vi "UHR-Fleezers Control (fpga) FB changed Ronen - 10.3.vi"() -> ()   [LabVIEW 2013]
doc: "UHR-Fleezers Instrument Control Code (fpga)"
uses:
  <vilib>/eio/EIONode/EIONode.xnode
  <vilib>/eio/EIOMethodNode/EIOMethodNode.xnode
  <vilib>/rvi/DataTransferAndStorage/Container/XNode/niFpgaContainer.xnode
  <vilib>/Platform/TimedLoop/XDataNode/XDataNode.xnode
  <vilib>/Platform/TimedLoop/XDataNode/nitl_modes.ctl
  <vilib>/Platform/TimedLoop/XDataNode/XDNodeRunTimeDep.lvlib
  <vilib>/Platform/TimedLoop/XDataNode/wakeup.ctl
  <vilib>/Platform/TimedLoop/XDataNode/timing_clust.ctl
  <vilib>/addons/control/pid/fpga.llb/XNode/niFpgaPID.xnode
  <vilib>/rvi/eio/common/nirviEmuTemplateMethod_errors.vi
  <vilib>/rvi/interface/RandomDataEmulation/nirviRandomDataFpgaReadWriteTemplate.vi
panel:
  out "Trap Pos FB Int-Norm Signal":fxp<+/-,24,9> format="%.16g"
  out "Trap Pos FB Int Signal":fxp<+/-,24,9> format="%.18g"
  in  "Tab Control":T1(tab)
  in  "AI1 X Scale":u16
  in  "Trap Pos FB Monitor T1 or T2":bool
  in  "Trap Pos FB Negate Action":bool
  in  "Trap Pos. FB SP":fxp<+/-,16,1>
  in  "Trap Pos. FB Reset":bool
  in  "Trap Pos to FIFO":bool
  in  "AI1 Sets to FIFO":T2={"Set 1"=TRUE, "Set 2"=TRUE, "Set 3"=FALSE}
  in  "N of AI1 Int Acq Sets":i16=2 min=1 max=3 step=1
  out "AI Late Counter":u16
  in  "ai count":u32=400
  out "AI late?":bool
  in  "+ phase":bool
  in  "Phase count adjustment":i16
  out "Relative phase":i16
  in  "AI to FIFO":bool
  out "BD1 Frequency Out 1":u64
  out "BD1 Frequency Out 2":u64
  in  "Force feedback":bool
  out "AI1 X Set 1":fxp<+/-,16,1>
  in  "Trap Pos. FB Gains":T3={"proportional gain (Kc)"=0.0, "integral gain (Kc*Ts/Ti)"=10.0, "derivative gain (Kc*Td/Ts)"=0.0} {"proportional gain (Kc)" format="%.11g"; "integral gain (Kc*Ts/Ti)" format="%.11g"; "derivative gain (Kc*Td/Ts)" format="%.11g"}
  in  "Trap Pos. FB Range":T4={"output high"=0.999969482421875, "output low"=-1.0}
  in  "Trap Pos. FB Mult Factor":i64=2
  in  "Trap Pos. FB Offset Factor":i64
  out "AI1 X Set 2":fxp<+/-,16,1>
  out "Trap Pos FB Action":i64
  out "Trap Pos FIFO Timeout":u16
  out "Trap AI FIFO Timeout":u16
  in  "Trap FIFO Set Timeout":i32
  in  "Trap Pos FB Int Count":u16=100
  in  "Dynamic Force FB (Ronen)":bool
  in  "Tab Control 2":T5(tab)
  in  "FB Min Frequency":u64
  in  "FB Max Frequency":u64
  in  "Negate Diff?":bool
  in  "B factor":fxp<+/-,16,16>
  in  "Diff FB Measurement?":bool
  in  "Swap F1 and F2":bool
  in  "Freq or Amp switch first":bool=TRUE
  in  "Cont. Scan":bool
  in  "Abort scan":bool
  in  "Cycles per step":u64
  in  "Scan BD":bool
  in  "Number of scans":u16
  in  "Scan steps":u64
  in  "Scan freq.  increment":i64
  out "Scanning":bool
  in  "Start scan":bool
  in  "OSK Bd 1":bool
  in  "Reset Bd 1":bool
  in  "RD":bool
  in  "PMODE":bool
  in  "OSK Bd 2":bool
  in  "Reset Bd 2":bool
  in  "Direct RF Box \nCommunication":bool
  in  "Data BD 2":u8 format="%08b"
  in  "Data BD 1":u8 format="%08b"
  in  "Address":u8 format="%02x"
  in  "Update Data":bool
  in  "FPGA Controls\n RF Box":bool
  in  "Number Interlace Cycles":u8=2 min=1 max=3
  in  "Interlace Off Parameters":u8=1 min=1 max=3
  in  "Interlace ON/OFF":bool
  out "DIO Relative phase":i16
  in  "Phase count adjustment (DIO)":i16
  in  "+ phase (DIO)":bool
  out "DIO Late Counter":u16
  out "DIO Late?":bool
  in  "DIO count 1 (ticks)":u32=400
  in  "DIO count 2 (ticks)":u32=400
  in  "DIO count 3 (ticks)":u32=400
  out "AI4 Y Sum Set 2":i16
  out "AI4 Y Sum Set 1":i16
  in  "FB Gains Set 1":T6={"proportional gain (Kc)"=10, "integral gain (Kc*Ts/Ti)"=5, "derivative gain (Kc*Td/Ts)"=0}
  in  "FB Setpoint Set 1":i16 min=0 step=1
  in  "FB Reset Set 1":bool
  in  "FB On/Off Set 1":bool
  in  "FB Reset Set 2":bool
  in  "FB On/Off Set 2":bool
  in  "FB Setpoint Set 2":i16 min=0 step=1
  in  "FB Gains Set 2":T6={"proportional gain (Kc)"=10, "integral gain (Kc*Ts/Ti)"=5, "derivative gain (Kc*Td/Ts)"=0}
  in  "FB output range 2":cluster{"output high":i16, "output low":i16}={"output high"=3000, "output low"=0}
  in  "FB output range 1":cluster{"output high":i16, "output low":i16}={"output high"=3000, "output low"=0}
  out "Scan I":u64
  in  "Amp switch delay":u16=5
  in  "Freq switch delay":u16
  in  "BD 2 Amplitude 1":u16
  in  "BD 1 Amplitude 1":u16
  in  "BD 2 Frequency 1":u64
  in  "BD 1 Frequency 1":u64
  in  "BD 2 Amplitude 2":u16
  in  "BD 1 Amplitude 2":u16
  in  "BD 2 Frequency 2":u64
  in  "BD 1 Frequency 2":u64
  in  "BD 2 Amplitude 3":u16
  in  "BD 1 Amplitude 3":u16
  in  "BD 2 Frequency 3":u64
  in  "BD 1 Frequency 3":u64
  out "Numeric":i32
  out "AO2 2":i16
  out "AO1 2":i16
  in  "1D or 2D Scan?":bool
  in  "Abort scan (MCL)":bool
  in  "MCL Scan Axis":bool
  in  "Cont. Scan (MCL)":bool
  out "Scan I (MCL)":u64
  in  "Number of scans (MCL)":u16
  out "Scanning MCL":bool
  in  "Scan steps (MCL)":u64
  in  "Cycles per step (MCL)":u64
  in  "Scan freq.  increment (MCL)":i16
  in  "Start scan (MCL)":bool
  in  "AO2":i16
  in  "AO1":i16
  out "MCL Late Counter":u16
  out "MCL Late?":bool
  in  "MCL count":u32=800
  out "MCL Relative Phase":i16
  in  "Phase count adjustment (MCL)":i16
  in  "+ phase (MCL)":bool
  in  "APD Gate Operating Mode":u8 max=2 step=1
  in  "Invert APD Gate":bool
  in  "APD Gate OFF Count":u32=100
  in  "APD Gate ON Count":u32=300
  out "APD 1 Gate Late Counter":u16
  out "APD 1 Gate Late?":bool
  out "APD 1 Gate Relative Phase":i16
  in  "Phase count adjustment (APD 1 Gate)":i16
  in  "+ phase (APD 1 Gate)":bool
  out "APD 2 Counts 0":u32
  out "APD 2 Counts 1":u32
  out "APD 1 Counts 0":u32
  out "APD 1 Counts 1":u32
  out "APD1 out state":bool
  in  "APD 2 AO scale factor":i16=1
  in  "APD 1 AO scale factor":i16=1
  in  "APD to FIFO":bool
  in  "APD Acq Rate Count":u32=20000000
  out "APD Acq Late Counter":u16
  out "APD Acq Late?":bool
  out "APD Acq Relative Phase":i16
  in  "Phase Count Adjustment (APD Acq)":i16
  in  "+ phase (APD Acq)":bool
  in  "Phase count adjustment (APD 2 Gate)":i16
  out "APD 2 Gate Late Counter":u16
  out "APD 2 Gate Late?":bool
  out "APD 2 Gate Relative Phase":i16
  in  "+ phase (APD 2 Gate)":bool
  out "APD2 out state":bool
  in  "Green Filter Flipper":bool
  out "Green FB Signals":T7
  in  "Green FB Count":u32=1200
  out "Green Late Counter":u16
  out "Green FB Late?":bool
  out "Green FB Relative Phase":i16
  in  "Phase count adjustment (Green FB)":i16=10
  in  "+ phase (Green FB)":bool
  out "Green FB Sum":i16
  in  "Green int current ON count adj":u32=150
  in  "Current Out":u16=30000
  in  "Green FB On/Off":bool
  in  "Green FB Setpoint":i16=250 min=0 step=1
  in  "Green FB Gains":T6={"proportional gain (Kc)"=10, "integral gain (Kc*Ts/Ti)"=5, "derivative gain (Kc*Td/Ts)"=0}
  in  "Green FB Reset":bool
  in  "Operating Mode 2":u8=2 max=2 step=1
  in  "Invert GI 2":bool
  in  "Green interlace OFF count 2":u32=900
  in  "Green interlace ON count 2":u32=300
  out "GI Late Counter 2":u16
  out "GI Late? 2":bool
  out "GI Relative phase 2":i16
  in  "Phase count adjustment (GI) 2":i16=20
  in  "+ phase (GI) 2":bool
  in  "Green interlace OFF count":u32=100
  out "GI Relative phase":i16
  in  "Phase count adjustment (GI)":i16
  in  "+ phase (GI)":bool
  out "GI Late?":bool
  in  "Green interlace ON count":u32=300
  out "GI Late Counter":u16
  in  "Invert GI":bool
  in  "Operating Mode":u8 max=2 step=1
  in  "Chassis2/Mod4/AO1":u16
  # "Only one of these can be on\nat a time:"
  # "Raster Scan AOD"
  # "1 (X)"
  # "2 (Y)"
  # "IR Intensity Feedback (RF BD 1)"
  # "AO1 (Y)"
  # "2D"
  # "1D"
  # "AO2 (X)"
  # "APD AO for aligning"
  # "Detection Loop"
  # "Green fluorescent laser digital gate interlacing loop"
  # "0 Forced ON\n1 Forced OFF\n2 Interlacing"
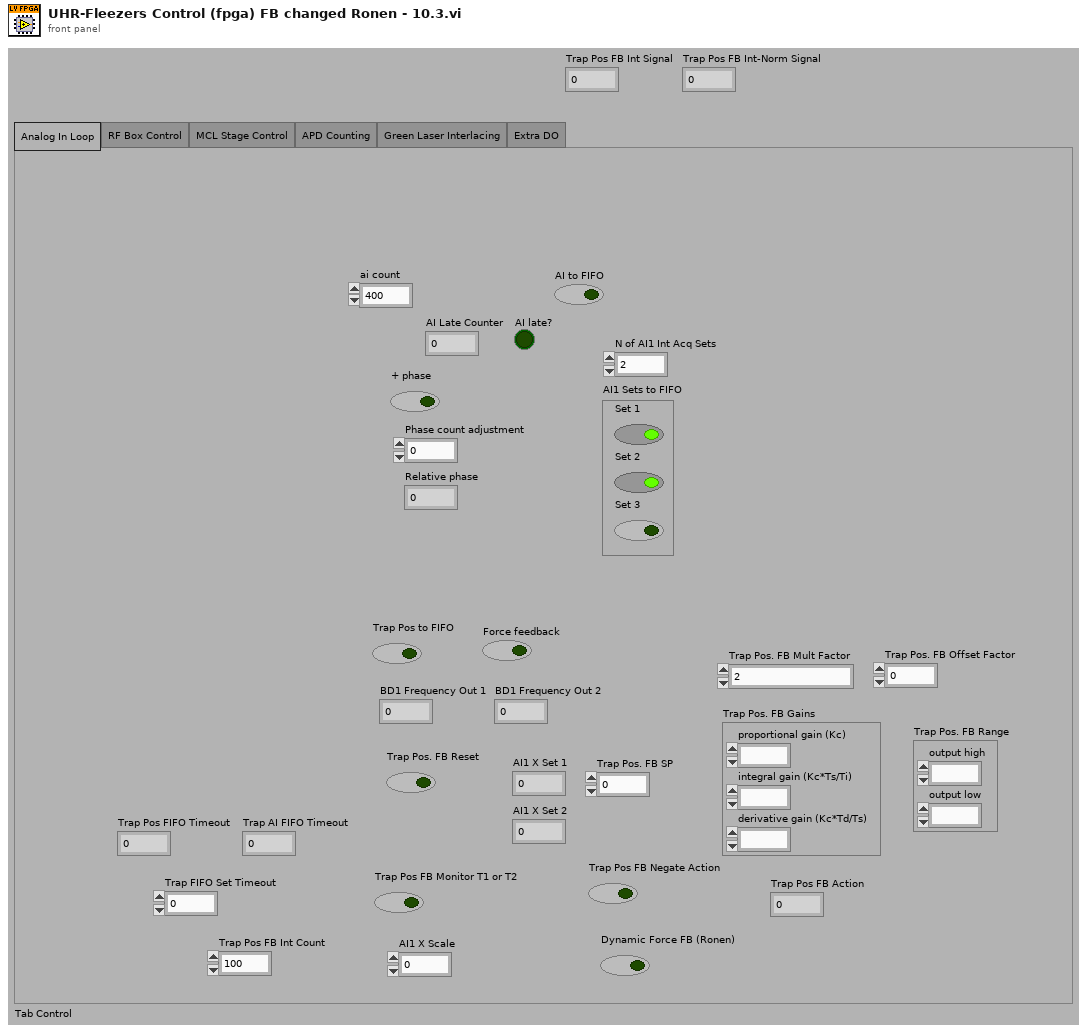
[diagram p1: front panel]
types:
  T1 = enum32{"Analog In Loop", "RF Box Control", "MCL Stage Control", "APD Counting", "Green Laser Interlacing", "Extra DO"}
  T2 = cluster{"Set 1":bool, "Set 2":bool, "Set 3":bool}
  T3 = cluster{"proportional gain (Kc)":fxp<+/-,16,8>, "integral gain (Kc*Ts/Ti)":fxp<+/-,16,8>, "derivative gain (Kc*Td/Ts)":fxp<+/-,16,8>}
  T4 = cluster{"output high":fxp<+/-,16,1>, "output low":fxp<+/-,16,1>}
  T5 = enum32{"Controls", "Interlacing Frequency and Amplitude Values"}
  T6 = cluster{"proportional gain (Kc)":i16, "integral gain (Kc*Ts/Ti)":i16, "derivative gain (Kc*Td/Ts)":i16}
  T7 = cluster{"Green FB Ch 0":i16, "Green FB Ch 1":i16, "Green FB Ch 2":i16}
  T8 = typedef "XDNodeRunTimeDep.lvlib/timing_clust.ctl" = cluster{"Expected End [f-1]":u64, "Actual End [f-1]":u64, "Finished Late? [f-1]":bool, "Expected End [i-1]":u64, "Actual End [i-1]":u64, "Finished Late? [i-1]":bool, "Expected Start [i]":u64, "Actual Start [i]":u64, "Expected Start [f]":u64, "Actual Start [f]":u64, "Source Name":string, "Structure Name":string, "Period":i64, "Deadline":i64, "Offset":i64, "Start":i64, "Priority":i32, "Timeout":i32, "Mode":T9, "Wakeup Reason":T10, "Error":errorcluster, "Source Type":string, "Secondary Source Type":string, "Global End Time":u64, "Global Start Time":u64, "Frame Duration":u64, "Iteration Duration":u64, "Assigned CPU":i32, "I/O Scan Engine Mode":u32}
  T9 = typedef "XDNodeRunTimeDep.lvlib/nitl_modes.ctl" = enum32{"No Change", "Process missed periods, maintain original phase", "Discard missed periods, maintain original phase", "Process missed periods, ignore original phase", "Discard missed periods, ignore original phase"}
  T10 = typedef "XDNodeRunTimeDep.lvlib/wakeup.ctl" = enum32{"Normal", "Aborted", "Asynchronous wakeup", "Timing source error", "Timed loop error", "Timeout"}
  T11 = cluster{"Chassis2/Mod2/AI0":i16, "Chassis2/Mod2/AI1":i16, "Chassis2/Mod2/AI2":i16}
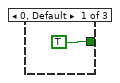
[diagram p2: hidden frame]
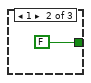
[diagram p3: hidden frame]
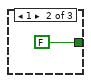
[diagram p5: hidden frame]
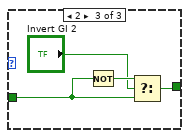
[diagram p6: hidden frame]
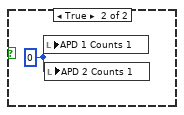
[diagram p7: hidden frame]
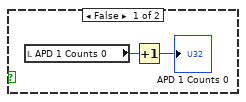
[diagram p9: hidden frame]
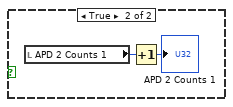
[diagram p10: hidden frame]
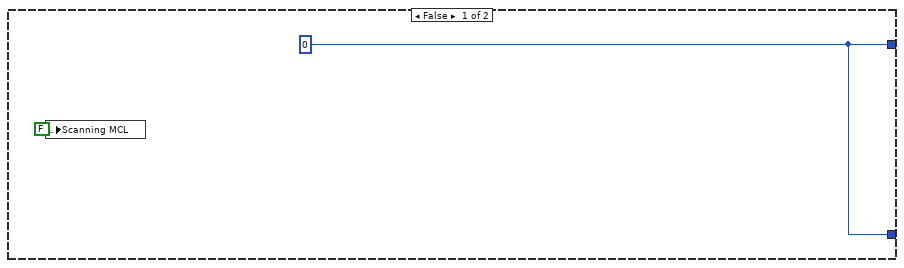
[diagram p11: hidden frame]
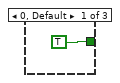
[diagram p12: hidden frame]
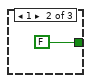
[diagram p13: hidden frame]
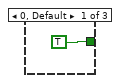
[diagram p14: hidden frame]
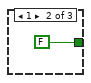
[diagram p15: hidden frame]
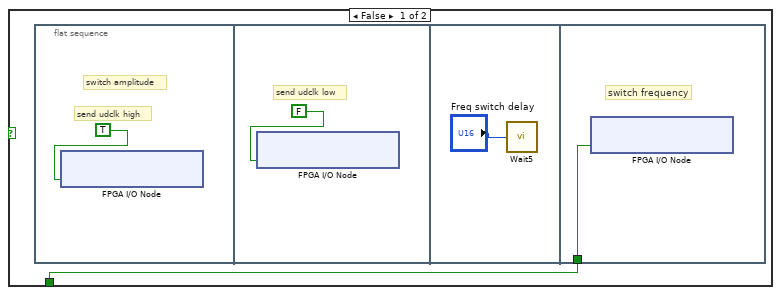
[diagram p18: hidden frame]
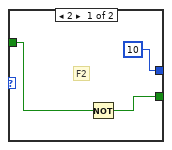
[diagram p20: hidden frame]
diagram:
  w4 = FALSE
  # "timing array current index"
  # "timing array"
  # "timing counter (phase adjusted here)"
  # "late counter"
  n1 = flat-sequence "FPGA initialization to do before running any of the loops" {
    tunnel: [u32 0 ("DIO count 3 (ticks)")] -> w3
    tunnel: [w11] -> _
    frame #0 {
      # "Start up expansion chassis early\nto avoid delays later"
      # "This pin controls udclk on the RF boards.\nWhen initially configuring the boards, this pin needs to be\nconfigured as a high impedance input.  Later it will be switched\nto an output."
      # "Initial setting of DIO data and \naddress to low (before reset).  \nThis needs to happen before the other\ncontrol method loops execute."
      n2 = xnode "FPGA I/O Node"("Connector1/DIO0"=FALSE, "Connector1/DIO1"=FALSE, "Connector1/DIO2"=FALSE, "Connector1/DIO3"=FALSE, "Connector1/DIO4"=FALSE, "Connector1/DIO5"=FALSE, "Connector1/DIO6"=FALSE, "Connector1/DIO7"=FALSE, "Connector1/DIO8"=FALSE, "Connector1/DIO9"=FALSE, "Connector1/DIO10"=FALSE, "Connector1/DIO11"=FALSE, "Connector1/DIO12"=FALSE, "Connector1/DIO13"=FALSE, "Connector1/DIO15"=FALSE, "Connector1/DIO20"=FALSE, "Connector1/DIO21"=FALSE, "Connector1/DIO22"=FALSE, "Connector1/DIO23"=FALSE, "Connector1/DIO24"=FALSE, "Connector1/DIO25"=FALSE, "Connector1/DIO26"=FALSE, "Connector1/DIO27"=FALSE, "Connector1/DIO14"=FALSE) -> ()  [unwired: 24 in, 24 out]
      n3 = xnode "FPGA I/O Method Node"("Enable"=FALSE) -> ()  [unwired: 1 in, 1 out]
      n4 = xnode "FPGA I/O Node"("Chassis2/Mod1/AO0"=u16 0 ("Chassis2/Mod4/AO0")) -> ("Chassis2/Mod2/AI0"=w11:i16)  [unwired: 2 in, 2 out]
    }
  }
  n5 = local read "AO1"() -> (w8:i16)
  n6 = local read "AO2"() -> (w7:i16)
  n7 = node-c288() -> (w6:T8)  [unwired: 1 in]
  n8 = while "APD 1 Counter" {
    tunnel: w3 -> [_]
    stop <- FALSE stop-if-true
    n9 = flat-sequence {
      frame #0 {
        n10 = xnode "FPGA I/O Method Node"("FPGA I/O In"=refnum<k21> "Connector0/DIO0" ("APD 1 DO"), "Timeout"=-1) -> ()  [unwired: 2 out]
      }
      frame #1 {
        n11 = local read "APD1 out state"() -> (w42:bool)
        n12 = case shown="True" w42 {
          frame False {
            n13 = local read "APD 1 Counts 0"() -> (w44:u32)
            n14 = Increment(x=w44) -> (x+1=→"APD 1 Counts 0":u32)
          }
          frame True {
            n15 = local read "APD 1 Counts 1"() -> (w46:u32)
            n16 = Increment(x=w46) -> (x+1=→"APD 1 Counts 1":u32)
          }
        }
      }
    }
  }
  n17 = while "APD 2 Counter" {
    tunnel: w3 -> [_]
    stop <- FALSE stop-if-true
    n18 = flat-sequence {
      frame #0 {
        n19 = xnode "FPGA I/O Method Node"("FPGA I/O In"=refnum<k21> "Connector0/DIO1" ("APD 2 DO"), "Timeout"=-1) -> ()  [unwired: 2 out]
      }
      frame #1 {
        n20 = local read "APD2 out state"() -> (w50:bool)
        n21 = case shown="False" w50 {
          frame False {
            n22 = local read "APD 2 Counts 0"() -> (w52:u32)
            n23 = Increment(x=w52) -> (x+1=→"APD 2 Counts 0":u32)
          }
          frame True {
            n24 = local read "APD 2 Counts 1"() -> (w54:u32)
            n25 = Increment(x=w54) -> (x+1=→"APD 2 Counts 1":u32)
          }
        }
      }
    }
  }
  n26 = timed-loop "RF box board DIO control: control bits" {
    timing: w6 -> [_]
    timing-out: [_] -> w5
    tunnel: [w55] -> _
    tunnel: w3 -> [w55]
    stop <- FALSE stop-if-true
    n27 = xnode "FPGA I/O Node"("Connector1/DIO16"="RD", "Connector1/DIO17"="PMODE", "Connector1/DIO18"="OSK Bd 1", "Connector1/DIO19"="Reset Bd 1", "Connector1/DIO28"="OSK Bd 2", "Connector1/DIO29"="Reset Bd 2") -> ()  [unwired: 6 in, 6 out]
  }
  n28 = while "Control Additional IO (Green laser flip mount)" {
    stop <- FALSE stop-if-true
    n29 = xnode "FPGA I/O Node"("Connector0/DIO3"="Green Filter Flipper", "Chassis2/Mod1/AO1"="Chassis2/Mod4/AO1") -> ()  [unwired: 2 in, 2 out]
    n30 = call "Loop Timer2"("Count(Ticks)"=u32 40000 ("Extra DO Counts")) -> ()  [unwired: 1 out]
  }
  n31 = while "RF box board direct communication loop" {
    tunnel: w3 -> [_]
    stop <- FALSE stop-if-true
    n32 = case "Whether to use direct communication method (only use one method at a time)" shown="True" "Direct RF Box \nCommunication" {
      frame False {
      }
      frame True {
        n33 = case shown="True" "Update Data" {
          frame False {
          }
          frame True {
            n34 = flat-sequence {
              frame #0 {
                n35 = First Call?() -> (First Call?: T/F=w72:bool)
                n36 = case shown="True" w72 {
                  frame False {
                  }
                  frame True {
                    # "If first time data updated, be sure to set WR high\nbefore setting data and address bits."
                    n37 = flat-sequence {
                      frame #0 {
                        n38 = xnode "FPGA I/O Node"("Connector1/DIO15"=TRUE) -> ()  [unwired: 1 in, 1 out]
                      }
                      frame #1 {
                        n39 = call "Wait"("Count(Ticks)"=u8 40 ("DO Delay 3 (Ticks)")) -> ()  [unwired: 1 out]
                      }
                    }
                  }
                }
              }
              frame #1 {
                n40 = Number To Boolean Array(number="Address") -> (Boolean array=w121:bool[])
                n41 = Number To Boolean Array(number="Data BD 1") -> (Boolean array=w122:bool[])
                n42 = Number To Boolean Array(number="Data BD 2") -> (Boolean array=w91:bool[])
                n43 = Index Array(array=w122, index=7) -> (element=w106:bool)
                n44 = Index Array(array=w122, index=6) -> (element=w105:bool)
                n45 = Index Array(array=w122, index=5) -> (element=w104:bool)
                n46 = Index Array(array=w122, index=4) -> (element=w103:bool)
                n47 = Index Array(array=w122, index=3) -> (element=w102:bool)
                n48 = Index Array(array=w122, index=2) -> (element=w101:bool)
                n49 = Index Array(array=w122, index=1) -> (element=w100:bool)
                n50 = Index Array(array=w122, index=0) -> (element=w99:bool)
                n51 = Index Array(array=w121, index=5) -> (element=w98:bool)
                n52 = Index Array(array=w121, index=4) -> (element=w97:bool)
                n53 = Index Array(array=w121, index=3) -> (element=w96:bool)
                n54 = Index Array(array=w121, index=2) -> (element=w95:bool)
                n55 = Index Array(array=w121, index=1) -> (element=w94:bool)
                n56 = Index Array(array=w121, index=0) -> (element=w93:bool)
                n57 = Index Array(array=w91, index=7) -> (element=w82:bool)
                n58 = Index Array(array=w91, index=6) -> (element=w81:bool)
                n59 = Index Array(array=w91, index=5) -> (element=w80:bool)
                n60 = Index Array(array=w91, index=4) -> (element=w79:bool)
                n61 = Index Array(array=w91, index=3) -> (element=w78:bool)
                n62 = Index Array(array=w91, index=2) -> (element=w77:bool)
                n63 = Index Array(array=w91, index=1) -> (element=w76:bool)
                n64 = Index Array(array=w91, index=0) -> (element=w75:bool)
                n65 = xnode "FPGA I/O Node"("Connector1/DIO0"=w106, "Connector1/DIO1"=w105, "Connector1/DIO2"=w104, "Connector1/DIO3"=w103, "Connector1/DIO4"=w102, "Connector1/DIO5"=w101, "Connector1/DIO6"=w100, "Connector1/DIO7"=w99, "Connector1/DIO8"=w98, "Connector1/DIO9"=w97, "Connector1/DIO10"=w96, "Connector1/DIO11"=w95, "Connector1/DIO12"=w94, "Connector1/DIO13"=w93, "Connector1/DIO20"=w82, "Connector1/DIO21"=w81, "Connector1/DIO22"=w80, "Connector1/DIO23"=w79, "Connector1/DIO24"=w78, "Connector1/DIO25"=w77, "Connector1/DIO26"=w76, "Connector1/DIO27"=w75) -> ()  [unwired: 22 in, 22 out]
              }
              frame #2 {
                # "wait and then apply write signal"
                n66 = call "Wait2"("Count(Ticks)"=u8 40 ("DO Delay 1 (Ticks)")) -> ()  [unwired: 1 out]
              }
              frame #3 {
                # "sending bit low writes data to board buffer"
                n67 = xnode "FPGA I/O Node"("Connector1/DIO15"=FALSE) -> ()  [unwired: 1 in, 1 out]
              }
              frame #4 {
                # "wait then return write signal"
                n68 = call "Wait3"("Count(Ticks)"=u8 40 ("DO Delay 2 (Ticks)")) -> ()  [unwired: 1 out]
              }
              frame #5 {
                # "sending bit high makes ready to\nwrite more data"
                n69 = xnode "FPGA I/O Node"("Connector1/DIO15"=TRUE) -> ()  [unwired: 1 in, 1 out]
              }
            }
          }
        }
      }
    }
  }
  n70 = while "APD 2 Gating" {
    shift-right: [w132] -> _
    shift-left: w3 -> [w137]
    shift-right: [w131] -> _
    shift-left: w4 -> [w129]
    stop <- FALSE stop-if-true
    n71 = flat-sequence {
      tunnel: w137 -> [w140]
      tunnel: [w141] -> w135
      tunnel: [w140] -> w133
      tunnel: [w139] -> w130
      tunnel: w129 -> [w139]
      tunnel: [w144] -> w136
      tunnel: w135 -> [w144]
      tunnel: [w143] -> w134
      tunnel: w133 -> [w143]
      tunnel: w130 -> [w142]
      tunnel: [w162] -> w132
      tunnel: w136 -> [w173]
      tunnel: w134 -> [w171]
      tunnel: [w166] -> w131
      frame #0 {
        n72 = call "Loop Timer8"("Count(Ticks)"=w140) -> ("Tick Count(Ticks)"=w141:u32)
      }
      frame #1 {
        # "(need 4 channels/APD)"
        n73 = xnode "FPGA I/O Node"("Connector1/DIO26"=w142, "Connector1/DIO27"=w142, "Connector1/DIO22"=w142, "Connector1/DIO32"=w142, "Connector1/DIO34"=w142, "Connector1/DIO33"=w142, "Connector1/DIO35"=w142) -> ()  [unwired: 7 in, 7 out]
      }
      frame #2 {
        n74 = local read "APD Gate ON Count"() -> (w155:u32)
        n75 = local read "APD Gate OFF Count"() -> (w154:u32)
        n76 = feedback #1(TRUE) -> (w168:bool)
        n77 = feedback-in #2(w173) -> ()
        n78 = feedback #2(w173) -> (w156:u32)
        n79 = Not(x=w168) -> (.not. x?=w165:bool)
        n80 = feedback-in #1(w165) -> ()
        n81 = Subtract(x=w173, y=w156) -> (x-y=w172:u32)
        n82 = Select(t=w155, s=w165, f=w154) -> (s? t:f=w170:u32)
        n83 = Subtract(x=w172, y=w171) -> (x-y=w147:u32)
        n84 = Subtract(x=w170, y=w147) -> (x-y=w161:u32)
        n85 = Number To Boolean Array(number=w147) -> (Boolean array=w146:bool[])
        n86 = Or Array Elements(Boolean array=w146) -> (logical OR=w145:bool)
        "APD 2 Gate Late?" <- w145
        n87 = Boolean To (0,1)(Boolean="+ phase (APD 2 Gate)") -> (0, 1=w159:i16)
        n88 = Multiply(x=w159, y="Phase count adjustment (APD 2 Gate)") -> (x*y=w157:i16)
        n89 = Boolean To (0,1)(Boolean=w145) -> (0, 1=w152:i16)
        n90 = Add(x=w161, y=w157) -> (x+y=w162:u32)
        n91 = To Unsigned Word Integer(number=w152) -> (unsigned 16bit integer=w149:u16)
        n92 = feedback #3(i16 0) -> (w164:i16)
        n93 = Subtract(x=w164, y=w157) -> (x-y=w163:i16)
        "APD 2 Gate Relative Phase" <- w163
        n94 = feedback-in #3(w163) -> ()
        n95 = feedback #4(u16 0) -> (w150:u16)
        n96 = Add(x=w149, y=w150) -> (x+y=w148:u16)
        "APD 2 Gate Late Counter" <- w148
        n97 = feedback-in #4(w148) -> ()
        n98 = local read "APD Gate Operating Mode"() -> (w153:u8)
        n99 = case shown="2" w153 {
          tunnel: [TRUE FALSE w179] -> w166
          tunnel: w168 -> [_ _ w177]
          frame 0, Default {
          }
          frame 1 {
          }
          frame 2 {
            n100 = local read "Invert APD Gate"() -> (w176:bool)
            n101 = Not(x=w177) -> (.not. x?=w178:bool)
            n102 = Select(t=w178, s=w176, f=w177) -> (s? t:f=w179:bool)
          }
        }
      }
    }
  }
  n103 = while "APD 1 Gating" {
    shift-right: [w183] -> _
    shift-left: w3 -> [w188]
    shift-right: [w182] -> _
    shift-left: w4 -> [w180]
    stop <- FALSE stop-if-true
    n104 = flat-sequence {
      tunnel: w188 -> [w191]
      tunnel: [w192] -> w186
      tunnel: [w191] -> w184
      tunnel: [w190] -> w181
      tunnel: w180 -> [w190]
      tunnel: [w195] -> w187
      tunnel: w186 -> [w195]
      tunnel: [w194] -> w185
      tunnel: w184 -> [w194]
      tunnel: w181 -> [w193]
      tunnel: [w209] -> w183
      tunnel: w187 -> [w224]
      tunnel: w185 -> [w221]
      tunnel: [w213] -> w182
      frame #0 {
        n105 = call "Loop Timer7"("Count(Ticks)"=w191) -> ("Tick Count(Ticks)"=w192:u32)
      }
      frame #1 {
        # "(need 4 channels/APD)"
        n106 = xnode "FPGA I/O Node"("Connector0/DIO8"=w193, "Connector0/DIO9"=w193, "Connector0/DIO10"=w193, "Connector0/DIO11"=w193, "Connector0/DIO4"=w193, "Connector0/DIO5"=w193, "Connector0/DIO6"=w193, "Connector0/DIO7"=w193) -> ()  [unwired: 8 in, 8 out]
      }
      frame #2 {
        n107 = feedback #5(TRUE) -> (w216:bool)
        n108 = feedback-in #6(w224) -> ()
        n109 = feedback #6(w224) -> (w223:u32)
        n110 = Not(x=w216) -> (.not. x?=w212:bool)
        n111 = feedback-in #5(w212) -> ()
        n112 = Subtract(x=w224, y=w223) -> (x-y=w222:u32)
        n113 = Select(t="APD Gate ON Count", s=w212, f="APD Gate OFF Count") -> (s? t:f=w218:u32)
        n114 = Subtract(x=w222, y=w221) -> (x-y=w197:u32)
        n115 = Subtract(x=w218, y=w197) -> (x-y=w208:u32)
        n116 = Number To Boolean Array(number=w197) -> (Boolean array=w198:bool[])
        n117 = Or Array Elements(Boolean array=w198) -> (logical OR=w196:bool)
        "APD 1 Gate Late?" <- w196
        n118 = Boolean To (0,1)(Boolean="+ phase (APD 1 Gate)") -> (0, 1=w206:i16)
        n119 = Boolean To (0,1)(Boolean=w196) -> (0, 1=w203:i16)
        n120 = Multiply(x=w206, y="Phase count adjustment (APD 1 Gate)") -> (x*y=w204:i16)
        n121 = To Unsigned Word Integer(number=w203) -> (unsigned 16bit integer=w200:u16)
        n122 = Add(x=w208, y=w204) -> (x+y=w209:u32)
        n123 = feedback #7(i16 0) -> (w211:i16)
        n124 = Subtract(x=w211, y=w204) -> (x-y=w210:i16)
        "APD 1 Gate Relative Phase" <- w210
        n125 = feedback-in #7(w210) -> ()
        n126 = feedback #8(u16 0) -> (w201:u16)
        n127 = Add(x=w200, y=w201) -> (x+y=w199:u16)
        "APD 1 Gate Late Counter" <- w199
        n128 = feedback-in #8(w199) -> ()
        n129 = case shown="2" "APD Gate Operating Mode" {
          tunnel: [TRUE FALSE w230] -> w213
          tunnel: w216 -> [_ _ w227]
          frame 0, Default {
          }
          frame 1 {
          }
          frame 2 {
            n130 = Not(x=w227) -> (.not. x?=w229:bool)
            n131 = Select(t=w229, s="Invert APD Gate", f=w227) -> (s? t:f=w230:bool)
          }
        }
      }
    }
  }
  n132 = while "DAQ AI set 1" {
    shift-right: [w231] -> _
    shift-left: w3 -> [w236]
    stop <- FALSE stop-if-true
    n133 = flat-sequence {
      tunnel: w236 -> [w246]
      tunnel: [w247] -> w234
      tunnel: [w246] -> w233
      tunnel: [w257] -> w244
      tunnel: [w256] -> w243
      tunnel: [w255] -> w242
      tunnel: [w254] -> w241
      tunnel: [w253] -> w240
      tunnel: [w252] -> w239
      tunnel: [w251] -> w238
      tunnel: [w250] -> w237
      tunnel: [w249] -> w235
      tunnel: w234 -> [w249]
      tunnel: w233 -> [w248]
      tunnel: [w248] -> w232
      tunnel: [w287] -> w231
      tunnel: w244 -> [w314]
      tunnel: w243 -> [w279]
      tunnel: w242 -> [w280]
      tunnel: w241 -> [w313]
      tunnel: w240 -> [w259]
      tunnel: w239 -> [w302]
      tunnel: w238 -> [w301]
      tunnel: w237 -> [w300]
      tunnel: w235 -> [w297]
      tunnel: w232 -> [w294]
      frame #0 {
        n134 = call "Loop Timer3"("Count(Ticks)"=w246) -> ("Tick Count(Ticks)"=w247:u32)
      }
      frame #1 {
        # "detection \nlaser qpd"
        # "sum"
        # "x"
        # "y"
        # "1064 int\nfeedback qpd"
        # "sum"
        # "x"
        # "traps\nqpd"
        # "sum"
        # "y"
        # "x"
        n135 = xnode "FPGA I/O Node"("Connector1/DIO31"=TRUE ("Connector1/DIO33")) -> ("Connector0/AI0"=w257:i16, "Connector0/AI1"=w256:i16, "Connector0/AI2"=w255:i16, "Connector0/AI3"=w254:i16, "Connector0/AI4"=w253:i16, "Connector0/AI5"=w252:i16, "Connector0/AI6"=w251:i16, "Connector0/AI7"=w250:i16)  [unwired: 9 in, 9 out]
      }
      frame #2 {
        w283 = FALSE ("AI to FIFO")
        # "only write specified sets (1 and 2 usually) to FIFO \nif AI to FIFO is true"
        # "Adjust phase after data acquired if button pressed"
        n136 = feedback #9(i16 1) -> (w306:i16)
        n137 = Increment(x=w306) -> (x+1=w312:i16)
        n138 = Scale By Power Of 2(n="AI1 X Scale", x=w279) -> (x*2^n=w277:i16)
        n139 = Greater?(x=w312, y="N of AI1 Int Acq Sets") -> (0:w309:bool)
        n140 = Divide(x=w277, y=w280) -> (x/y=w276:fxp<+/-,16,1>)
        n141 = Select(t=i16 1, s=w309, f=w312) -> (s? t:f=w311:i16)
        n142 = feedback-in #9(w311) -> ()
        n143 = feedback #10(w283) -> (w281:bool)
        n144 = feedback #11(w283) -> (w299:bool)
        n145 = case shown="3" w306 {
          tunnel: w259 -> [w336 w344 _]
          tunnel: "AI1 Sets to FIFO" -> [w340 w348 w354]
          tunnel: [w339 w347 w353] -> w303
          tunnel: ["AI to FIFO" w346 w352] -> w298
          tunnel: w299 -> [_ w346 w352]
          tunnel: ["Trap Pos to FIFO" w345 w351] -> w282
          tunnel: w281 -> [_ w345 w351]
          tunnel: w276 -> [w335 w343 _]
          tunnel: [w334 w341 FALSE] -> w263
          tunnel: [w333 w342 u64 0 ("BD1 Frequency Out 2")] -> w262
          frame 1, Default {
            n146 = Unbundle By Name(w340) -> ("Set 1"=w339:bool)
            n147 = local read "BD1 Frequency Out 1"() -> (w333:u64)
            n148 = Compound Arithmetic op=AND("Trap Pos to FIFO", w339, "AI to FIFO") -> (w334:bool)
            "AI4 Y Sum Set 1" <- w336
            "AI1 X Set 1" <- w335
          }
          frame 2 {
            n149 = Unbundle By Name(w348) -> ("Set 2"=w347:bool)
            n150 = local read "BD1 Frequency Out 2"() -> (w342:u64)
            n151 = Compound Arithmetic op=AND(w345, w347, w346) -> (w341:bool)
            "AI4 Y Sum Set 2" <- w344
            "AI1 X Set 2" <- w343
          }
          frame 3 {
            n152 = Unbundle By Name(w354) -> ("Set 3"=w353:bool)
          }
        }
        n153 = And(x=w303, y=w298) -> (x .and. y?=w305:bool)
        n154 = feedback-in #10(w282) -> ()
        n155 = case shown="True" w305 {
          tunnel: w314 -> [_ w368]
          tunnel: w279 -> [_ w367]
          tunnel: w280 -> [_ w366]
          tunnel: w313 -> [_ w365]
          tunnel: w259 -> [_ w364]
          tunnel: w302 -> [_ w363]
          tunnel: w301 -> [_ w362]
          tunnel: w300 -> [_ w361]
          tunnel: 0 ("DMA buffer timeout") -> [_ w370]
          frame False {
          }
          frame True {
            n156 = Build Array(w368, w367, w366, w365, w364, w363, w362, w361) -> (w369:i16[])
            n157 = for {
              tunnel: w369 -> [w372] mode=indexing
              tunnel: w370 -> [w373]
              tunnel: [w371] -> w359 mode=indexing
              n158 = xnode ("FIFO Write")("Element"=w372, "Timeout"=w373) -> ("Timed Out?"=w371:bool)  [unwired: 1 in, 1 out]
            }
            n159 = Or Array Elements(Boolean array=w359) -> (logical OR=w356:bool)
            n160 = Boolean To (0,1)(Boolean=w356) -> (0, 1=w358:i16)
            n161 = feedback #12(u16 0) -> (w357:u16)
            n162 = Add(x=w358, y=w357) -> (x+y=w355:u16)
            "Trap AI FIFO Timeout" <- w355
            n163 = feedback-in #12(w355) -> ()
          }
        }
        n164 = feedback-in #11(w298) -> ()
        n165 = case shown="True" w263 {
          tunnel: w262 -> [_ w320]
          tunnel: [u8 0 w317] -> w261
          frame False {
          }
          frame True {
            n166 = Split Number(x=w320) -> (hi(x)=w321:u32, lo(x)=w322:u32)
            n167 = Split Number(x=w321) -> (lo(x)=w323:u16)  [unwired: 1 out]
            n168 = Split Number(x=w322) -> (hi(x)=w324:u16, lo(x)=w325:u16)
            n169 = Build Array "BD 1 nu Stack"(w323, w324, w325) -> (w319:u16[])
            n170 = for {
              tunnel: w319 -> [w332] mode=indexing
              shift-right: [w328] -> w317
              shift-left: u8 0 -> [w329]
              n171 = xnode ("FIFO Method Node")("Element"=w332, "Timeout"="Trap FIFO Set Timeout") -> ("Timed Out?"=w331:bool)  [unwired: 1 in, 1 out]
              n172 = Boolean To (0,1)(Boolean=w331) -> (0, 1=w330:i16)
              n173 = To Unsigned Byte Integer(number=w330) -> (unsigned 8bit integer=w327:u8)
              n174 = Add(x=w327, y=w329) -> (x+y=w328:u8)
            }
          }
        }
        n175 = To Unsigned Word Integer(number=w261) -> (unsigned 16bit integer=w260:u16)
        n176 = feedback #13(u16 0) -> (w274:u16)
        n177 = Add(x=w260, y=w274) -> (x+y=w273:u16)
        "Trap Pos FIFO Timeout" <- w273
        n178 = feedback-in #13(w273) -> ()
        n179 = feedback-in #14(w297) -> ()
        n180 = feedback #14(w297) -> (w296:u32)
        n181 = Subtract(x=w297, y=w296) -> (x-y=w295:u32)
        n182 = xnode "I/O Node"("Connector1/DIO31"=FALSE ("Connector1/DIO34")) -> ()  [unwired: 1 in, 1 out]
        n183 = Subtract(x=w295, y=w294) -> (x-y=w265:u32)
        n184 = Boolean To (0,1)(Boolean="+ phase") -> (0, 1=w290:i16)
        n185 = Multiply(x=w290, y="Phase count adjustment") -> (x*y=w284:i16)
        n186 = Subtract(x="ai count", y=w265) -> (x-y=w288:u32)
        n187 = Number To Boolean Array(number=w265) -> (Boolean array=w266:bool[])
        n188 = feedback #15(i16 0) -> (w286:i16)
        n189 = Add(x=w288, y=w284) -> (x+y=w287:u32)
        n190 = Subtract(x=w286, y=w284) -> (x-y=w285:i16)
        "Relative phase" <- w285
        n191 = feedback-in #15(w285) -> ()
        n192 = Or Array Elements(Boolean array=w266) -> (logical OR=w264:bool)
        "AI late?" <- w264
        n193 = Boolean To (0,1)(Boolean=w264) -> (0, 1=w271:i16)
        n194 = To Unsigned Word Integer(number=w271) -> (unsigned 16bit integer=w268:u16)
        n195 = feedback #16(u16 0) -> (w269:u16)
        n196 = Add(x=w268, y=w269) -> (x+y=w267:u16)
        "AI Late Counter" <- w267
        n197 = feedback-in #16(w267) -> ()
      }
    }
  }
  n198 = while "MCL stage control" {
    shift-right: [w389] -> _
    shift-left: w3 -> [w392]
    shift-right: [w382] -> _
    shift-left: w8 -> [w379]
    shift-right: [w381] -> _
    shift-left: w7 -> [w377]
    i -> [w376]
    stop <- FALSE stop-if-true
    n199 = flat-sequence {
      tunnel: w392 -> [w396]
      tunnel: [w397] -> w388
      tunnel: [w396] -> w386
      tunnel: [w395] -> w380
      tunnel: w379 -> [w395]
      tunnel: [w394] -> w378
      tunnel: w377 -> [w394]
      tunnel: w388 -> [w401]
      tunnel: [w401] -> w387
      tunnel: w386 -> [w400]
      tunnel: [w400] -> w385
      tunnel: w380 -> [w399]
      tunnel: w378 -> [w398]
      tunnel: [w399] -> w375
      tunnel: [w398] -> w374
      tunnel: w387 -> [w411]
      tunnel: w385 -> [w410]
      tunnel: [w411] -> w391
      tunnel: [w410] -> w390
      tunnel: [w409] -> w384
      tunnel: [w408] -> w383
      tunnel: w375 -> [w403]
      tunnel: w374 -> [w402]
      tunnel: [w483] -> w389
      tunnel: w391 -> [w490]
      tunnel: w390 -> [w487]
      tunnel: w384 -> [w485]
      tunnel: w383 -> [w484]
      tunnel: [w485] -> w382
      tunnel: [w484] -> w381
      frame #0 {
        n200 = call "Loop Timer5"("Count(Ticks)"=w396) -> ("Tick Count(Ticks)"=w397:u32)
      }
      frame #1 {
        n201 = xnode "FPGA I/O Node"("Connector0/AO1"=w399, "Connector0/AO2"=w398) -> ()  [unwired: 2 in, 2 out]
      }
      frame #2 {
        n202 = local read "Scanning MCL"() -> (w423:bool)
        n203 = Or(x=w423, y="Start scan (MCL)") -> (x .or. y?=w418:bool)
        n204 = Not(x="Abort scan (MCL)") -> (.not. x?=w416:bool)
        n205 = And(x=w416, y=w418) -> (x .and. y?=w415:bool)
        n206 = case "Raster scan" shown="True" w415 {
          tunnel: [w424 w467] -> w420
          tunnel: "Start scan (MCL)" -> [_ w452]
          tunnel: [w424 w428] -> w404
          frame False {
            w424 = i16 0
            n207 = local write "Scanning MCL"(FALSE ("scanning")) -> ()
          }
          frame True {
            w438 = i16 0
            w437 = u64 0
            # "scan incr."
            # "freq. incr. mult."
            # "count steps"
            # "count number of cycles"
            n208 = feedback #17(w437) -> (w464:u64)
            n209 = Select(t=w437, s=w452, f=w464) -> (s? t:f=w466:u64)
            n210 = Increment(x=w466) -> (x+1=w463:u64)
            n211 = Greater?(x="Cycles per step (MCL)", y=w463) -> (0:w447:bool)
            n212 = Select(t=w463, s=w447, f=w437) -> (s? t:f=w462:u64)
            n213 = feedback-in #17(w462) -> ()
            n214 = feedback #18(w437) -> (w461:u64)
            n215 = Select(t=w437, s=w452, f=w461) -> (s? t:f=w456:u64)
            n216 = Increment(x=w456) -> (x+1=w460:u64)
            n217 = Add(x="Scan steps (MCL)", y="Scan steps (MCL)") -> (x+y=w459:u64)
            n218 = Select(t=w456, s=w447, f=w460) -> (s? t:f=w442:u64)
            n219 = Greater?(x=w459, y=w442) -> (0:w441:bool)
            n220 = Select(t=w442, s=w441, f=w437) -> (s? t:f=w457:u64)
            n221 = feedback-in #18(w457) -> ()
            n222 = Equal?(x="Scan steps (MCL)", y=w442) -> (x = y?=w446:bool)
            n223 = Greater?(x="Scan steps (MCL)", y=w456) -> (0:w455:bool)
            n224 = feedback #19(w438) -> (w458:i16)
            n225 = Select(t=w438, s=w452, f=w458) -> (s? t:f=w444:i16)
            n226 = Increment(x=w444) -> (x+1=w454:i16)
            n227 = Decrement(x=w444) -> (x-1=w453:i16)
            n228 = Select(t=w454, s=w455, f=w453) -> (s? t:f=w445:i16)
            n229 = Select(t=w444, s=w446, f=w445) -> (s? t:f=w443:i16)
            n230 = Select(t=w444, s=w447, f=w443) -> (s? t:f=w439:i16)
            n231 = Select(t=w439, s=w441, f=w438) -> (s? t:f=w440:i16)
            n232 = feedback-in #19(w440) -> ()
            n233 = feedback #20(w437) -> (w451:u64)
            n234 = Select(t=w437, s=w452, f=w451) -> (s? t:f=w426:u64)
            n235 = Increment(x=w426) -> (x+1=w448:u64)
            n236 = Select(t=w426, s=w441, f=w448) -> (s? t:f=w427:u64)
            n237 = Greater?(x="Number of scans (MCL)", y=w427) -> (0:w434:bool)
            n238 = Multiply(x="Scan freq.  increment (MCL)", y=w444) -> (x*y=w467:i16)
            n239 = Select(t=TRUE, s="Cont. Scan (MCL)", f=w434) -> (s? t:f=w433:bool)
            "Scanning MCL" <- w433
            n240 = Select(t=w427, s=w433, f=w437) -> (s? t:f=w449:u64)
            n241 = feedback-in #20(w449) -> ()
            n242 = Increment(x=w427) -> (x+1=→"Scan I (MCL)":u64)
            n243 = To Word Integer(number=w426) -> (16bit integer=w429:i16)
            n244 = Multiply(x=w429, y="Scan freq.  increment (MCL)") -> (x*y=w428:i16)
          }
        }
        n245 = Select(t=w404, s="1D or 2D Scan?", f=i16 0) -> (s? t:f=w405:i16)
        n246 = Select(t=w405, s="MCL Scan Axis", f=w420) -> (s? t:f=w419:i16)
        n247 = Select(t=w420, s="MCL Scan Axis", f=w405) -> (s? t:f=w421:i16)
        n248 = Add(x=w419, y="AO2") -> (x+y=w408:i16)
        n249 = Add(x="AO1", y=w421) -> (x+y=w409:i16)
        "AO1 2" <- w403
        "AO2 2" <- w402
      }
      frame #3 {
        n250 = feedback-in #21(w490) -> ()
        n251 = feedback #21(w490) -> (w489:u32)
        n252 = Boolean To (0,1)(Boolean="+ phase (MCL)") -> (0, 1=w481:i16)
        n253 = Subtract(x=w490, y=w489) -> (x-y=w488:u32)
        n254 = Multiply(x=w481, y="Phase count adjustment (MCL)") -> (x*y=w477:i16)
        n255 = Subtract(x=w488, y=w487) -> (x-y=w469:u32)
        n256 = Subtract(x="MCL count", y=w469) -> (x-y=w479:u32)
        n257 = feedback #22(i16 0) -> (w478:i16)
        n258 = Subtract(x=w478, y=w477) -> (x-y=w476:i16)
        "MCL Relative Phase" <- w476
        n259 = feedback-in #22(w476) -> ()
        n260 = Number To Boolean Array(number=w469) -> (Boolean array=w470:bool[])
        n261 = Or Array Elements(Boolean array=w470) -> (logical OR=w468:bool)
        "MCL Late?" <- w468
        n262 = Boolean To (0,1)(Boolean=w468) -> (0, 1=w475:i16)
        n263 = Add(x=w479, y=w477) -> (x+y=w483:u32)
        n264 = To Unsigned Word Integer(number=w475) -> (unsigned 16bit integer=w472:u16)
        n265 = feedback #23(u16 0) -> (w473:u16)
        n266 = Add(x=w472, y=w473) -> (x+y=w471:u16)
        "MCL Late Counter" <- w471
        n267 = feedback-in #23(w471) -> ()
      }
    }
    "Numeric" <- w376
  }
  n268 = while "Control APD data integration - stream to host" {
    shift-right: [w494] -> _
    shift-left: w3 -> [w499]
    stop <- FALSE stop-if-true
    n269 = flat-sequence {
      tunnel: w499 -> [w501]
      tunnel: [w502] -> w497
      tunnel: [w501] -> w495
      tunnel: [w510] -> w498
      tunnel: w497 -> [w510]
      tunnel: [w509] -> w496
      tunnel: w495 -> [w509]
      tunnel: [w508] -> w493
      tunnel: [w507] -> w492
      tunnel: [w544] -> w494
      tunnel: w498 -> [w556]
      tunnel: w496 -> [w553]
      tunnel: w493 -> [w537]
      tunnel: w492 -> [w536]
      frame #0 {
        n270 = call "Loop Timer6"("Count(Ticks)"=w501) -> ("Tick Count(Ticks)"=w502:u32)
      }
      frame #1 {
        n271 = flat-sequence {
          tunnel: [w512] -> w506
          tunnel: w506 -> [w514]
          tunnel: [w516] -> w505
          tunnel: [w515] -> w504
          tunnel: [w514] -> w503
          tunnel: [w522] -> w507
          tunnel: [w523] -> w508
          tunnel: w505 -> [w523]
          tunnel: w504 -> [w522]
          tunnel: w503 -> [w521]
          frame #0 {
            # "use two separate variable so each APD won't\nhave to wait to read"
            n272 = feedback #24(FALSE) -> (w511:bool)
            "APD1 out state" <- w511
            "APD2 out state" <- w511
            n273 = Not(x=w511) -> (.not. x?=w512:bool)
            n274 = feedback-in #24(w512) -> ()
          }
          frame #1 {
            n275 = local read "APD 1 Counts 1"() -> (w520:u32)
            n276 = local read "APD 1 Counts 0"() -> (w519:u32)
            n277 = local read "APD 2 Counts 1"() -> (w518:u32)
            n278 = local read "APD 2 Counts 0"() -> (w517:u32)
            n279 = Select(t=w520, s=w514, f=w519) -> (s? t:f=w516:u32)
            n280 = Select(t=w518, s=w514, f=w517) -> (s? t:f=w515:u32)
          }
          frame #2 {
            n281 = case shown="False" w521 {
              frame False {
                w524 = u32 0 ("APD 1 Counts 0")
                n282 = local write "APD 1 Counts 0"(w524) -> ()
                n283 = local write "APD 2 Counts 0"(w524) -> ()
              }
              frame True {
                w525 = u32 0 ("APD 1 Counts 1")
                n284 = local write "APD 1 Counts 1"(w525) -> ()
                n285 = local write "APD 2 Counts 1"(w525) -> ()
              }
            }
          }
        }
      }
      frame #2 {
        n286 = feedback-in #25(w556) -> ()
        n287 = feedback #25(w556) -> (w555:u32)
        n288 = Subtract(x=w556, y=w555) -> (x-y=w554:u32)
        n289 = Subtract(x=w554, y=w553) -> (x-y=w529:u32)
        n290 = case shown="True" "APD to FIFO" {
          tunnel: w537 -> [_ w559]
          tunnel: w536 -> [_ w557]
          frame False {
          }
          frame True {
            n291 = flat-sequence {
              tunnel: 0 ("Timeout") -> [w561]
              tunnel: w559 -> [w562]
              tunnel: [w561] -> w558
              tunnel: w558 -> [w564]
              tunnel: w557 -> [w563]
              frame #0 {
                n292 = xnode ("FIFO Write")("Element"=w562, "Timeout"=w561) -> ()  [unwired: 1 in, 2 out]
              }
              frame #1 {
                n293 = xnode ("FIFO Write")("Element"=w563, "Timeout"=w564) -> ()  [unwired: 1 in, 2 out]
              }
            }
          }
        }
        n294 = Subtract(x="APD Acq Rate Count", y=w529) -> (x-y=w545:u32)
        n295 = Number To Boolean Array(number=w529) -> (Boolean array=w530:bool[])
        n296 = Or Array Elements(Boolean array=w530) -> (logical OR=w528:bool)
        "APD Acq Late?" <- w528
        n297 = Boolean To (0,1)(Boolean=w528) -> (0, 1=w535:i16)
        n298 = To Unsigned Word Integer(number=w535) -> (unsigned 16bit integer=w532:u16)
        n299 = Boolean To (0,1)(Boolean="+ phase (APD Acq)") -> (0, 1=w541:i16)
        n300 = feedback #26(u16 0) -> (w533:u16)
        n301 = Add(x=w532, y=w533) -> (x+y=w531:u16)
        "APD Acq Late Counter" <- w531
        n302 = feedback-in #26(w531) -> ()
        n303 = Multiply(x=w541, y="Phase Count Adjustment (APD Acq)") -> (x*y=w538:i16)
        n304 = Add(x=w545, y=w538) -> (x+y=w544:u32)
        n305 = feedback #27(i16 0) -> (w543:i16)
        n306 = Subtract(x=w543, y=w538) -> (x-y=w540:i16)
        "APD Acq Relative Phase" <- w540
        n307 = feedback-in #27(w540) -> ()
        n308 = To Word Integer(number=w537) -> (16bit integer=w546:i16)
        n309 = To Word Integer(number=w536) -> (16bit integer=w547:i16)
        n310 = Multiply(x="APD 1 AO scale factor", y=w546) -> (x*y=w527:i16)
        n311 = Multiply(x="APD 2 AO scale factor", y=w547) -> (x*y=w526:i16)
        n312 = xnode "FPGA I/O Node"("Connector0/AO6"=w527, "Connector0/AO7"=w526) -> ()  [unwired: 2 in, 2 out]
      }
    }
  }
  n313 = while "Green fluorescent laser interlacing (DO to IA 532 nm AOM ME amp)." {
    shift-right: [w568] -> _
    shift-left: w3 -> [w573]
    shift-right: [w567] -> _
    shift-left: FALSE -> [w565]
    stop <- FALSE stop-if-true
    n314 = flat-sequence {
      tunnel: w573 -> [w576]
      tunnel: [w577] -> w571
      tunnel: [w576] -> w569
      tunnel: [w575] -> w566
      tunnel: w565 -> [w575]
      tunnel: [w580] -> w572
      tunnel: w571 -> [w580]
      tunnel: [w579] -> w570
      tunnel: w569 -> [w579]
      tunnel: w566 -> [w578]
      tunnel: [w589] -> w568
      tunnel: w572 -> [w609]
      tunnel: w570 -> [w606]
      tunnel: [w598] -> w567
      frame #0 {
        n315 = call "Loop Timer4"("Count(Ticks)"=w576) -> ("Tick Count(Ticks)"=w577:u32)
      }
      frame #1 {
        n316 = xnode "FPGA I/O Node"("Connector1/DIO37"=w578, "Connector1/DIO38"=w578, "Connector1/DIO39"=w578) -> ()  [unwired: 3 in, 3 out]
      }
      frame #2 {
        n317 = feedback-in #28(w609) -> ()
        n318 = feedback #28(w609) -> (w608:u32)
        n319 = Subtract(x=w609, y=w608) -> (x-y=w607:u32)
        n320 = Subtract(x=w607, y=w606) -> (x-y=w582:u32)
        n321 = Number To Boolean Array(number=w582) -> (Boolean array=w583:bool[])
        n322 = Or Array Elements(Boolean array=w583) -> (logical OR=w581:bool)
        "GI Late?" <- w581
        n323 = Boolean To (0,1)(Boolean="+ phase (GI)") -> (0, 1=w594:i16)
        n324 = Multiply(x=w594, y="Phase count adjustment (GI)") -> (x*y=w591:i16)
        n325 = Boolean To (0,1)(Boolean=w581) -> (0, 1=w588:i16)
        n326 = To Unsigned Word Integer(number=w588) -> (unsigned 16bit integer=w585:u16)
        n327 = feedback #29(i16 0) -> (w592:i16)
        n328 = feedback #30(u16 0) -> (w586:u16)
        n329 = Add(x=w585, y=w586) -> (x+y=w584:u16)
        "GI Late Counter" <- w584
        n330 = feedback-in #30(w584) -> ()
        n331 = Subtract(x=w592, y=w591) -> (x-y=w590:i16)
        "GI Relative phase" <- w590
        n332 = feedback-in #29(w590) -> ()
        n333 = feedback #31(TRUE) -> (w601:bool)
        n334 = case shown="2" "Operating Mode" {
          tunnel: [TRUE FALSE w615] -> w598
          tunnel: w601 -> [_ _ w612]
          frame 0, Default {
          }
          frame 1 {
          }
          frame 2 {
            n335 = Not(x=w612) -> (.not. x?=w614:bool)
            n336 = Select(t=w614, s="Invert GI", f=w612) -> (s? t:f=w615:bool)
          }
        }
        n337 = Not(x=w601) -> (.not. x?=w597:bool)
        n338 = Select(t="Green interlace ON count", s=w597, f="Green interlace OFF count") -> (s? t:f=w603:u32)
        n339 = Subtract(x=w603, y=w582) -> (x-y=w595:u32)
        n340 = Add(x=w595, y=w591) -> (x+y=w589:u32)
        n341 = feedback-in #31(w597) -> ()
      }
    }
  }
  n342 = while "Green fluorescent laser interlacing (Current to IA 532 nm AOM ME amp)." {
    shift-right: [w621] -> _
    shift-left: w3 -> [w624]
    shift-right: [w618] -> _
    shift-left: u16 0 -> [w616]
    stop <- FALSE stop-if-true
    n343 = flat-sequence {
      tunnel: w624 -> [w627]
      tunnel: [w628] -> w623
      tunnel: [w627] -> w622
      tunnel: [w626] -> w617
      tunnel: w616 -> [w626]
      tunnel: [w631] -> w620
      tunnel: w623 -> [w631]
      tunnel: [w630] -> w619
      tunnel: w622 -> [w630]
      tunnel: w617 -> [w629]
      tunnel: [w640] -> w621
      tunnel: [w657] -> w618
      tunnel: w620 -> [w670]
      tunnel: w619 -> [w667]
      frame #0 {
        n344 = call "Loop Timer10"("Count(Ticks)"=w627) -> ("Tick Count(Ticks)"=w628:u32)
      }
      frame #1 {
        n345 = xnode "FPGA I/O Node"("Chassis2/Mod1/AO0"=w629) -> ()  [unwired: 1 in, 1 out]
      }
      frame #2 {
        n346 = Subtract(x="Green interlace OFF count 2", y="Green int current ON count adj") -> (x-y=w649:u32)
        n347 = feedback-in #32(w670) -> ()
        n348 = feedback #32(w670) -> (w669:u32)
        n349 = Add(x="Green int current ON count adj", y="Green interlace ON count 2") -> (x+y=w650:u32)
        n350 = Subtract(x=w670, y=w669) -> (x-y=w668:u32)
        n351 = Subtract(x=w668, y=w667) -> (x-y=w633:u32)
        n352 = Number To Boolean Array(number=w633) -> (Boolean array=w634:bool[])
        n353 = Boolean To (0,1)(Boolean="+ phase (GI) 2") -> (0, 1=w646:i16)
        n354 = Or Array Elements(Boolean array=w634) -> (logical OR=w632:bool)
        "GI Late? 2" <- w632
        n355 = Boolean To (0,1)(Boolean=w632) -> (0, 1=w639:i16)
        n356 = Multiply(x=w646, y="Phase count adjustment (GI) 2") -> (x*y=w642:i16)
        n357 = To Unsigned Word Integer(number=w639) -> (unsigned 16bit integer=w635:u16)
        n358 = feedback #33(u16 0) -> (w637:u16)
        n359 = Add(x=w635, y=w637) -> (x+y=w636:u16)
        "GI Late Counter 2" <- w636
        n360 = feedback-in #33(w636) -> ()
        n361 = feedback #34(i16 0) -> (w643:i16)
        n362 = Subtract(x=w643, y=w642) -> (x-y=w641:i16)
        "GI Relative phase 2" <- w641
        n363 = feedback-in #34(w641) -> ()
        n364 = feedback #35(TRUE) -> (w662:bool)
        n365 = case shown="0, Default" "Operating Mode 2" {
          tunnel: [TRUE FALSE w687] -> w651
          tunnel: w662 -> [_ _ w684]
          frame 0, Default {
          }
          frame 1 {
          }
          frame 2 {
            n366 = Not(x=w684) -> (.not. x?=w686:bool)
            n367 = Select(t=w686, s="Invert GI 2", f=w684) -> (s? t:f=w687:bool)
          }
        }
        n368 = And(x=w651, y="Green FB On/Off") -> (x .and. y?=w652:bool)
        n369 = case shown="True" w652 {
          tunnel: "Current Out" -> [w671 _]
          tunnel: [w671 w676] -> w656
          frame False {
          }
          frame True {
            n370 = local read "Green FB Sum"() -> (w672:i16)
            n371 = call "Slower PID.vi"("process variable"=w672, "reset?"="Green FB Reset", "setpoint"="Green FB Setpoint", "PID gains (x 2^8)"="Green FB Gains", "output range"=cluster{"output high":i16, "output low":i16} {"output high"=32767, "output low"=-32768} ("Green FB output range")) -> ("output"=w680:i16)  [unwired: 10 out]
            n372 = To Long Integer(number=w680) -> (32bit integer=w673:i32)
            n373 = Add(x=w673, y=32768) -> (x+y=w675:i32)
            n374 = To Unsigned Word Integer(number=w675) -> (unsigned 16bit integer=w676:u16)
          }
        }
        n375 = Not(x=w662) -> (.not. x?=w659:bool)
        n376 = Select(t=w650, s=w659, f=w649) -> (s? t:f=w664:u32)
        n377 = Subtract(x=w664, y=w633) -> (x-y=w644:u32)
        n378 = Add(x=w644, y=w642) -> (x+y=w640:u32)
        n379 = feedback-in #35(w659) -> ()
        n380 = Boolean To (0,1)(Boolean=w651) -> (0, 1=w658:i16)
        n381 = To Unsigned Word Integer(number=w658) -> (unsigned 16bit integer=w655:u16)
        n382 = Multiply(x=w655, y=w656) -> (x*y=w657:u16)
      }
    }
  }
  n383 = while "Green excitation laser feedback measurement" {
    shift-right: [w688] -> _
    shift-left: w3 -> [w693]
    stop <- FALSE stop-if-true
    n384 = flat-sequence {
      tunnel: w693 -> [w695]
      tunnel: [w696] -> w691
      tunnel: [w695] -> w689
      tunnel: [w703] -> w692
      tunnel: w691 -> [w703]
      tunnel: [w702] -> w690
      tunnel: w689 -> [w702]
      tunnel: [w715] -> w688
      tunnel: w692 -> [w726]
      tunnel: w690 -> [w723]
      frame #0 {
        n385 = call "Loop Timer9"("Count(Ticks)"=w695) -> ("Tick Count(Ticks)"=w696:u32)
      }
      frame #1 {
        n386 = xnode "FPGA I/O Node"("Connector1/DIO35"=TRUE) -> ("Chassis2/Mod2/AI0"=w701:i16, "Chassis2/Mod2/AI1"=w700:i16, "Chassis2/Mod2/AI2"=w697:i16)  [unwired: 4 in, 4 out]
        "Green FB Sum" <- w697
        n387 = Bundle("Chassis2/Mod2/AI0"=w701, "Chassis2/Mod2/AI1"=w700, "Chassis2/Mod2/AI2"=w697) -> (→"Green FB Signals":T11)  [unwired: 1 out]
      }
      frame #2 {
        n388 = feedback-in #36(w726) -> ()
        n389 = feedback #36(w726) -> (w725:u32)
        n390 = Subtract(x=w726, y=w725) -> (x-y=w724:u32)
        n391 = xnode "FPGA I/O Node"("Connector1/DIO35"=FALSE) -> ()  [unwired: 1 in, 1 out]
        n392 = Subtract(x=w724, y=w723) -> (x-y=w705:u32)
        n393 = Subtract(x="Green FB Count", y=w705) -> (x-y=w719:u32)
        n394 = Number To Boolean Array(number=w705) -> (Boolean array=w706:bool[])
        n395 = Or Array Elements(Boolean array=w706) -> (logical OR=w704:bool)
        "Green FB Late?" <- w704
        n396 = Boolean To (0,1)(Boolean="+ phase (Green FB)") -> (0, 1=w717:i16)
        n397 = Boolean To (0,1)(Boolean=w704) -> (0, 1=w711:i16)
        n398 = Multiply(x=w717, y="Phase count adjustment (Green FB)") -> (x*y=w712:i16)
        n399 = Add(x=w719, y=w712) -> (x+y=w715:u32)
        n400 = To Unsigned Word Integer(number=w711) -> (unsigned 16bit integer=w708:u16)
        n401 = feedback #37(i16 0) -> (w714:i16)
        n402 = Subtract(x=w714, y=w712) -> (x-y=w713:i16)
        "Green FB Relative Phase" <- w713
        n403 = feedback-in #37(w713) -> ()
        n404 = feedback #38(u16 0) -> (w709:u16)
        n405 = Add(x=w708, y=w709) -> (x+y=w707:u16)
        "Green Late Counter" <- w707
        n406 = feedback-in #38(w707) -> ()
      }
    }
  }
  n407 = while "RF box board DIO control: parallel communication" {
    shift-right: [w735] -> _
    shift-left: w3 -> [w734]
    shift-right: [w733] -> _
    shift-left: FALSE ("Swap F1 and F2") -> [w732]
    shift-right: [w728] -> _
    shift-left: u64 0 -> [w727]
    stop <- FALSE stop-if-true
    n408 = flat-sequence {
      tunnel: w732 -> [w739]
      tunnel: w734 -> [w737]
      tunnel: [w739] -> w731
      tunnel: [w738] -> w730
      tunnel: [w737] -> w729
      tunnel: [w747] -> w735
      tunnel: [w746] -> w733
      tunnel: w731 -> [w745]
      tunnel: w730 -> [w743]
      tunnel: w729 -> [w742]
      tunnel: [w741] -> w728
      tunnel: w727 -> [w740]
      frame #0 {
        n409 = call "Loop Timer"("Count(Ticks)"=w737) -> ("Tick Count(Ticks)"=w738:u32)
      }
      frame #1 {
        n410 = flat-sequence {
          tunnel: ["FPGA Controls\n RF Box"] -> w744
          tunnel: w745 -> [w748]
          tunnel: [w790] -> w747
          tunnel: [w803] -> w746
          tunnel: w744 -> [w802]
          tunnel: w743 -> [w796]
          tunnel: w742 -> [w793]
          tunnel: [w769] -> w741
          tunnel: w740 -> [w768]
          frame #0 {
            n411 = case shown="True" "FPGA Controls\n RF Box" {
              tunnel: w748 -> [_ w750]
              frame False {
              }
              frame True {
                n412 = flat-sequence {
                  tunnel: w750 -> [w756]
                  frame #0 {
                    n413 = First Call?() -> (First Call?: T/F=w751:bool)
                    n414 = case shown="True" w751 {
                      frame False {
                      }
                      frame True {
                        # "If first time data updated, be sure to set WR high and UDCLK low\nbefore setting data and address bits."
                        n415 = xnode "FPGA I/O Method Node"("Enable"=TRUE) -> ("FPGA I/O Out"=w753:refnum<k21>)  [unwired: 1 in]
                        n416 = xnode "FPGA I/O Node"("Connector1/DIO15"=TRUE) -> ()  [unwired: 1 in, 1 out]
                        n417 = xnode "FPGA I/O Node"("I/O Item"=FALSE ("Connector1/DIO30"), "FPGA I/O In"=w753) -> ()  [unwired: 1 out]
                      }
                    }
                  }
                  frame #1 {
                    n418 = case shown="True" "Freq or Amp switch first" {
                      tunnel: w756 -> [w758 w763]
                      frame False {
                        n419 = flat-sequence {
                          tunnel: w758 -> [w762]
                          frame #0 {
                            # "switch amplitude"
                            # "send udclk high"
                            n420 = xnode "FPGA I/O Node"("Connector1/DIO30"=TRUE ("Connector1/DIO15")) -> ()  [unwired: 1 in, 1 out]
                          }
                          frame #1 {
                            # "send udclk low"
                            n421 = xnode "FPGA I/O Node"("Connector1/DIO30"=FALSE ("Connector1/DIO15")) -> ()  [unwired: 1 in, 1 out]
                          }
                          frame #2 {
                            n422 = call "Wait5"("Count(Ticks)"="Freq switch delay") -> ()  [unwired: 1 out]
                          }
                          frame #3 {
                            # "switch frequency"
                            n423 = xnode "FPGA I/O Node"("Connector1/DIO36"=w762) -> ()  [unwired: 1 in, 1 out]
                          }
                        }
                      }
                      frame True {
                        n424 = flat-sequence {
                          tunnel: w763 -> [w764]
                          frame #0 {
                            # "switch frequency"
                            n425 = xnode "FPGA I/O Node"("Connector1/DIO36"=w764) -> ()  [unwired: 1 in, 1 out]
                          }
                          frame #1 {
                            n426 = call "Wait4"("Count(Ticks)"="Amp switch delay") -> ()  [unwired: 1 out]
                          }
                          frame #2 {
                            # "switch amplitude"
                            # "send udclk high"
                            n427 = xnode "FPGA I/O Node"("Connector1/DIO30"=TRUE ("Connector1/DIO15")) -> ()  [unwired: 1 in, 1 out]
                          }
                          frame #3 {
                            # "send udclk low"
                            n428 = xnode "FPGA I/O Node"("Connector1/DIO30"=FALSE ("Connector1/DIO15")) -> ()  [unwired: 1 in, 1 out]
                          }
                        }
                      }
                    }
                  }
                }
              }
            }
          }
          frame #1 {
            # "This is the prior cycle's on time"
            # "increment timing\nindex, reset to 0 if \nend of matrix"
            # "Reset to begginning (1) when number of cycles reached."
            # "timing index"
            # "build byte stacks for writing data\n(must correspond to addresses array constant)"
            # "Timing housekeeping"
            # "Adjust phase if late\n(maintains constant phase relationship between cycles)"
            n429 = feedback #39(u8 0 ("t")) -> (w799:u8)
            n430 = Increment(x=w799) -> (x+1=w843:u8)
            n431 = Increment(x="Number Interlace Cycles") -> (x+1=w838:u8)
            n432 = Equal?(x=w843, y=w838) -> (x = y?=w845:bool)
            n433 = Select(t=u8 1, s=w845, f=w843) -> (s? t:f=w798:u8)
            n434 = feedback-in #39(w798) -> ()
            n435 = Increment(x=w798) -> (x+1=w840:u8)
            n436 = Equal?(x=w840, y=w838) -> (x = y?=w841:bool)
            n437 = Select(t=u8 1, s=w841, f=w840) -> (s? t:f=w837:u8)
            n438 = Select(t=w837, s="Interlace ON/OFF", f="Interlace Off Parameters") -> (s? t:f=w821:u8)
            n439 = case shown="1, Default" w821 {
              tunnel: [w882 "BD 1 Frequency 2" "BD 1 Frequency 3"] -> w833
              tunnel: [w924 "BD 2 Frequency 2" "BD 2 Frequency 3"] -> w822
              tunnel: ["BD 2 Amplitude 1" "BD 2 Amplitude 2" "BD 2 Amplitude 3"] -> w778
              tunnel: [w913 w1061 "BD 1 Amplitude 3"] -> w781
              tunnel: [w882 w1058 w1073] -> w769
              tunnel: w768 -> [w885 w1058 w1073]
              frame 1, Default {
                w901 = fxp<+/-,24,9> 0.0 ("AI1 X Set 2")
                w906 = u16 0
                w920 = u64 0 ("f")
                # "Trap 1"
                n440 = local read "AI1 X Set 2"() -> (w911:fxp<+/-,16,1>)
                n441 = local read "AI1 X Set 1"() -> (w909:fxp<+/-,16,1>)
                n442 = local read "Scanning"() -> (w925:bool)
                n443 = Multiply(x=w911, y="B factor") -> (x*y=w910:fxp<+/-,32,17>)
                n444 = feedback #40(w906) -> (w905:u16)
                n445 = Increment(x=w905) -> (x+1=w907:u16)
                n446 = case shown="True" "Diff FB Measurement?" {
                  tunnel: w910 -> [w943 w954]
                  tunnel: w909 -> [w944 w953]
                  tunnel: [w941 w945] -> w904
                  frame False {
                    n447 = Select(t=w944, s="Trap Pos FB Monitor T1 or T2", f=w943) -> (s? t:f=w941:fxp<+/-,32,17>)
                  }
                  frame True {
                    n448 = Subtract(x=w953, y=w954) -> (x-y=w952:fxp<+/-,32,17>)
                    n449 = Not(x="Negate Diff?") -> (.not. x?=w950:bool)
                    n450 = Boolean To (0,1)(Boolean="Negate Diff?") -> (0, 1=w948:i16)
                    n451 = Boolean To (0,1)(Boolean=w950) -> (0, 1=w949:i16)
                    n452 = Negate(x=w948) -> (-x=w947:i16)
                    n453 = Add(x=w947, y=w949) -> (x+y=w946:i16)
                    n454 = Multiply(x=w946, y=w952) -> (x*y=w945:fxp<+/-,47,32>)
                  }
                }
                n455 = Or(x=w925, y="Start scan") -> (x .or. y?=w918:bool)
                n456 = Greater Or Equal?(x=w907, y="Trap Pos FB Int Count") -> (x >= y?=w888:bool)
                n457 = Select(t=w906, s=w888, f=w907) -> (s? t:f=w908:u16)
                n458 = feedback-in #40(w908) -> ()
                n459 = Not(x="Abort scan") -> (.not. x?=w916:bool)
                n460 = And(x=w916, y=w918) -> (x .and. y?=w915:bool)
                n461 = case "For raster scanning" shown="True" w915 {
                  tunnel: [u64 0 w1048] -> w921
                  tunnel: "Start scan" -> [_ w1033]
                  frame False {
                    n462 = local write "Scanning"(FALSE ("scanning")) -> ()
                  }
                  frame True {
                    w1017 = i64 0
                    w1016 = u64 0
                    # "scan incr."
                    # "freq. incr. mult."
                    # "count steps"
                    # "count number of cycles"
                    n463 = feedback #41(w1016) -> (w1045:u64)
                    n464 = Select(t=w1016, s=w1033, f=w1045) -> (s? t:f=w1047:u64)
                    n465 = Increment(x=w1047) -> (x+1=w1044:u64)
                    n466 = Greater?(x="Cycles per step", y=w1044) -> (0:w1026:bool)
                    n467 = Select(t=w1044, s=w1026, f=w1016) -> (s? t:f=w1043:u64)
                    n468 = feedback-in #41(w1043) -> ()
                    n469 = feedback #42(w1016) -> (w1042:u64)
                    n470 = Select(t=w1016, s=w1033, f=w1042) -> (s? t:f=w1037:u64)
                    n471 = Increment(x=w1037) -> (x+1=w1041:u64)
                    n472 = Add(x="Scan steps", y="Scan steps") -> (x+y=w1040:u64)
                    n473 = Select(t=w1037, s=w1026, f=w1041) -> (s? t:f=w1021:u64)
                    n474 = Greater?(x=w1040, y=w1021) -> (0:w1020:bool)
                    n475 = Select(t=w1021, s=w1020, f=w1016) -> (s? t:f=w1038:u64)
                    n476 = feedback-in #42(w1038) -> ()
                    n477 = Equal?(x="Scan steps", y=w1021) -> (x = y?=w1025:bool)
                    n478 = Greater?(x="Scan steps", y=w1037) -> (0:w1036:bool)
                    n479 = feedback #43(w1017) -> (w1039:i64)
                    n480 = Select(t=w1017, s=w1033, f=w1039) -> (s? t:f=w1023:i64)
                    n481 = Increment(x=w1023) -> (x+1=w1035:i64)
                    n482 = Decrement(x=w1023) -> (x-1=w1034:i64)
                    n483 = Select(t=w1035, s=w1036, f=w1034) -> (s? t:f=w1024:i64)
                    n484 = Select(t=w1023, s=w1025, f=w1024) -> (s? t:f=w1022:i64)
                    n485 = Select(t=w1023, s=w1026, f=w1022) -> (s? t:f=w1018:i64)
                    n486 = Select(t=w1018, s=w1020, f=w1017) -> (s? t:f=w1019:i64)
                    n487 = feedback-in #43(w1019) -> ()
                    n488 = feedback #44(w1016) -> (w1032:u64)
                    n489 = Select(t=w1016, s=w1033, f=w1032) -> (s? t:f=w1028:u64)
                    n490 = Increment(x=w1028) -> (x+1=w1029:u64)
                    n491 = Select(t=w1028, s=w1020, f=w1029) -> (s? t:f=w1027:u64)
                    n492 = Greater?(x="Number of scans", y=w1027) -> (0:w1013:bool)
                    n493 = Multiply(x="Scan freq.  increment", y=w1023) -> (x*y=w1048:i64)
                    n494 = Select(t=TRUE, s="Cont. Scan", f=w1013) -> (s? t:f=w1012:bool)
                    "Scanning" <- w1012
                    n495 = Select(t=w1027, s=w1012, f=w1016) -> (s? t:f=w1030:u64)
                    n496 = feedback-in #44(w1030) -> ()
                    n497 = Increment(x=w1027) -> (x+1=→"Scan I":u64)
                  }
                }
                n498 = feedback #45(w901) -> (w902:fxp<+/-,24,9>)
                n499 = Add(x=w904, y=w902) -> (x+y=w895:fxp<+/-,24,9>)
                n500 = Select(t=w901, s=w888, f=w895) -> (s? t:f=w903:fxp<+/-,24,9>)
                n501 = feedback-in #45(w903) -> ()
                n502 = feedback #46(fxp<+/-,24,9> 0.0 ("AI1 X Set 2")) -> (w899:fxp<+/-,24,9>)
                n503 = Select(t=w895, s=w888, f=w899) -> (s? t:f=w896:fxp<+/-,24,9>)
                "Trap Pos FB Int Signal" <- w896
                n504 = feedback-in #46(w896) -> ()
                n505 = Divide(x=w895, y="Trap Pos FB Int Count") -> (x/y=w893:fxp<+/-,16,1>)
                n506 = case "For intensity feedback" shown="True" "FB On/Off Set 1" {
                  tunnel: "BD 1 Amplitude 1" -> [w1050 _]
                  tunnel: [w1050 w1051] -> w913
                  frame False {
                  }
                  frame True {
                    n507 = local read "AI4 Y Sum Set 1"() -> (w1053:i16)
                    n508 = call "Slower PID.vi"("process variable"=w1053, "reset?"="FB Reset Set 1", "setpoint"="FB Setpoint Set 1", "PID gains (x 2^8)"="FB Gains Set 1", "output range"="FB output range 1") -> ("output"=w1056:i16)  [unwired: 10 out]
                    n509 = To Unsigned Word Integer(number=w1056) -> (unsigned 16bit integer=w1051:u16)
                  }
                }
                n510 = feedback #47(fxp<+/-,24,9> 0.0 ("AI1 X Set 2")) -> (w897:fxp<+/-,24,9>)
                n511 = Select(t=w893, s=w888, f=w897) -> (s? t:f=w892:fxp<+/-,24,9>)
                "Trap Pos FB Int-Norm Signal" <- w892
                n512 = feedback-in #47(w892) -> ()
                n513 = case "For position feedback" shown="True" "Force feedback" {
                  tunnel: [i64 0 w960] -> w887
                  tunnel: w888 -> [_ w957]
                  tunnel: w893 -> [_ w956]
                  frame False {
                  }
                  frame True {
                    n514 = feedback #48(i64 0) -> (w959:i64)
                    n515 = case shown="True" w957 {
                      tunnel: [w961 w973] -> w960
                      tunnel: w959 -> [w961 _]
                      tunnel: w956 -> [_ w962]
                      frame False {
                      }
                      frame True {
                        n516 = xnode ("PID")("process variable"=w962, "reset?"="Trap Pos. FB Reset", "setpoint"="Trap Pos. FB SP", "PID gains"="Trap Pos. FB Gains", "output range"="Trap Pos. FB Range") -> ("output"=w971:fxp<+/-,16,1>)
                        n517 = Negate(x=w971) -> (-x=w970:fxp<+/-,17,2>)
                        n518 = Select(t=w970, s="Trap Pos FB Negate Action", f=w971) -> (s? t:f=w967:fxp<+/-,17,2>)
                        n519 = Scale By Power Of 2(n=u32 15, x=u32 1) -> (x*2^n=w964:u32)
                        n520 = Multiply(x=w967, y=w964) -> (x*y=w963:fxp<+/-,17,17>)
                        n521 = To Quad Integer(1:w963) -> (0:w976:i64)
                        "Trap Pos FB Action" <- w976
                        n522 = Multiply(x=w976, y="Trap Pos. FB Mult Factor") -> (x*y=w974:i64)
                        n523 = Add(x=w974, y="Trap Pos. FB Offset Factor") -> (x+y=w973:i64)
                      }
                    }
                    n524 = feedback-in #48(w960) -> ()
                  }
                }
                n525 = And(x="Force feedback", y="Dynamic Force FB (Ronen)") -> (x .and. y?=w889:bool)
                n526 = case shown="False" w889 {
                  tunnel: w888 -> [_ w936]
                  tunnel: w887 -> [w931 w935]
                  tunnel: [w930 w934] -> w886
                  tunnel: w885 -> [_ w933]
                  frame False {
                    n527 = Add(x="BD 1 Frequency 1", y=w931) -> (x+y=w930:u64)
                  }
                  frame True {
                    n528 = case shown="True" w936 {
                      tunnel: w935 -> [_ w940]
                      tunnel: [w937 w939] -> w934
                      tunnel: w933 -> [w937 w938]
                      frame False {
                      }
                      frame True {
                        n529 = Add(x=w940, y=w938) -> (x+y=w939:u64)
                      }
                    }
                  }
                }
                n530 = Select(t=w920, s="Scan BD", f=w921) -> (s? t:f=w919:u64)
                n531 = Select(t=w921, s="Scan BD", f=w920) -> (s? t:f=w922:u64)
                n532 = Add(x=w919, y="BD 2 Frequency 1") -> (x+y=w924:u64)
                n533 = Compound Arithmetic op=ADD(w886, i16 0, w922) -> (w883:u64)
                n534 = In Range and Coerce(upper limit="FB Max Frequency", x=w883, lower limit="FB Min Frequency") -> (coerced(x)=w882:u64)  [unwired: 1 out]
                "BD1 Frequency Out 1" <- w882
              }
              frame 2 {
                # "Trap 2"
                n535 = case shown="True" "FB On/Off Set 2" {
                  tunnel: [w1065 w1066] -> w1061
                  tunnel: "BD 1 Amplitude 2" -> [w1065 _]
                  frame False {
                  }
                  frame True {
                    n536 = local read "AI4 Y Sum Set 2"() -> (w1071:i16)
                    n537 = call "Slower PID.vi"("process variable"=w1071, "reset?"="FB Reset Set 2", "setpoint"="FB Setpoint Set 2", "PID gains (x 2^8)"="FB Gains Set 2", "output range"="FB output range 2") -> ("output"=w1068:i16)  [unwired: 10 out]
                    n538 = To Unsigned Word Integer(number=w1068) -> (unsigned 16bit integer=w1066:u16)
                  }
                }
                "BD1 Frequency Out 2" <- "BD 1 Frequency 2"
              }
              frame 3 {
                # "Fluorescence period"
              }
            }
            n539 = feedback-in #49(w796) -> ()
            n540 = feedback #49(w796) -> (w795:u32)
            n541 = Select(t=w798, s="Interlace ON/OFF", f="Interlace Off Parameters") -> (s? t:f=w836:u8)
            n542 = Subtract(x=w796, y=w795) -> (x-y=w794:u32)
            n543 = Subtract "The error"(x=w794, y=w793) -> (x-y=w771:u32)
            n544 = case shown="1, Default" w836 {
              tunnel: ["DIO count 1 (ticks)" "DIO count 2 (ticks)" "DIO count 3 (ticks)"] -> w792
              frame 1, Default {
              }
              frame 2 {
              }
              frame 3 {
              }
            }
            n545 = Number To Boolean Array(number=w771) -> (Boolean array=w772:bool[])
            n546 = Or Array Elements(Boolean array=w772) -> (logical OR=w770:bool)
            "DIO Late?" <- w770
            n547 = Boolean To (0,1)(Boolean=w770) -> (0, 1=w777:i16)
            n548 = To Unsigned Word Integer(number=w777) -> (unsigned 16bit integer=w774:u16)
            n549 = feedback #50(u16 0) -> (w775:u16)
            n550 = Add(x=w774, y=w775) -> (x+y=w773:u16)
            "DIO Late Counter" <- w773
            n551 = feedback-in #50(w773) -> ()
            n552 = Subtract(x=w792, y=w771) -> (x-y=w791:u32)
            n553 = Boolean To (0,1)(Boolean="+ phase (DIO)") -> (0, 1=w788:i16)
            n554 = Split Number(x=w778) -> (hi(x)=w780:u8, lo(x)=w779:u8)
            n555 = Multiply(x=w788, y="Phase count adjustment (DIO)") -> (x*y=w784:i16)
            n556 = feedback #51(i16 0) -> (w786:i16)
            n557 = Subtract(x=w786, y=w784) -> (x-y=w785:i16)
            "DIO Relative phase" <- w785
            n558 = feedback-in #51(w785) -> ()
            n559 = Add(x=w791, y=w784) -> (x+y=w790:u32)
            n560 = Build Array "BD 2 A Stack"(w780, w779) -> (w804:u8[])
            n561 = Split Number(x=w833) -> (hi(x)=w832:u32, lo(x)=w831:u32)
            n562 = Split Number(x=w822) -> (hi(x)=w827:u32, lo(x)=w826:u32)
            n563 = Split Number(x=w832) -> (lo(x)=w830:u16)  [unwired: 1 out]
            n564 = Split Number(x=w831) -> (hi(x)=w829:u16, lo(x)=w828:u16)
            n565 = Split Number(x=w827) -> (lo(x)=w825:u16)  [unwired: 1 out]
            n566 = Split Number(x=w826) -> (hi(x)=w824:u16, lo(x)=w823:u16)
            n567 = Split Number(x=w781) -> (hi(x)=w783:u8, lo(x)=w782:u8)
            n568 = Split Number(x=w830) -> (hi(x)=w820:u8, lo(x)=w819:u8)
            n569 = Split Number(x=w829) -> (hi(x)=w818:u8, lo(x)=w817:u8)
            n570 = Split Number(x=w825) -> (hi(x)=w813:u8, lo(x)=w812:u8)
            n571 = Split Number(x=w828) -> (hi(x)=w816:u8, lo(x)=w815:u8)
            n572 = Split Number(x=w824) -> (hi(x)=w811:u8, lo(x)=w810:u8)
            n573 = Split Number(x=w823) -> (hi(x)=w809:u8, lo(x)=w808:u8)
            n574 = Build Array "BD 1 A Stack"(w783, w782) -> (w805:u8[])
            n575 = Build Array "BD 1 nu Stack"(w820, w819, w818, w817, w816, w815) -> (w814:u8[])
            n576 = Build Array "BD 2 nu Stack"(w813, w812, w811, w810, w809, w808) -> (w807:u8[])
            n577 = case shown="1, Default" w821 {
              tunnel: [w871 w874] -> w803
              tunnel: [u8 10 u8 4] -> w806
              tunnel: "Swap F1 and F2" -> [w872 w874]
              frame 2 {
                # "F2"
                n578 = Not(x=w872) -> (.not. x?=w871:bool)
              }
              frame 1, Default {
                # "low chooses F1"
                # "F1"
              }
            }
            n579 = case "If FPGA is controlling (toggling) RF synth" shown="True" w802 {
              tunnel: w814 -> [_ w850]
              tunnel: w807 -> [_ w849]
              tunnel: w806 -> [_ w848]
              tunnel: w805 -> [_ w847]
              tunnel: w804 -> [_ w846]
              frame False {
              }
              frame True {
                # "Write next amp.\n(wait until beginning of next loop iteration to update)"
                n580 = flat-sequence "Update the next F1 and F2 frequency value (the actual frequency won't change until FSK is switched).\nThen load the next amplitude value into buffer, but don't update it until the next cycle." {
                  tunnel: w850 -> [w853]
                  tunnel: w849 -> [w852]
                  tunnel: w848 -> [w851]
                  tunnel: w847 -> [w864]
                  tunnel: w846 -> [w863]
                  frame #0 {
                    n581 = for {
                      tunnel: w853 -> [w859] mode=indexing
                      tunnel: w852 -> [w858] mode=indexing
                      tunnel: w851 -> [w856]
                      i -> [w857]
                      # "Write next freq."
                      n582 = To Unsigned Byte Integer(number=w857) -> (unsigned 8bit integer=w854:u8)
                      n583 = Add(x=w856, y=w854) -> (x+y=w855:u8)
                      n584 = call "write to RF synth bd.vi"("Address Byte"=w855, "BD 2 Byte"=w858, "BD 1 Byte"=w859) -> ()  [unwired: 2 in]
                    }
                  }
                  frame #1 {
                    # "send udclk high"
                    n585 = xnode "FPGA I/O Node"("Connector1/DIO30"=TRUE ("Connector1/DIO15")) -> ()  [unwired: 1 in, 1 out]
                  }
                  frame #2 {
                    n586 = xnode "FPGA I/O Node"("Connector1/DIO30"=FALSE ("Connector1/DIO15")) -> ()  [unwired: 1 in, 1 out]
                  }
                  frame #3 {
                    n587 = for {
                      tunnel: w864 -> [w870] mode=indexing
                      tunnel: w863 -> [w869] mode=indexing
                      tunnel: u8 33 -> [w867]
                      i -> [w868]
                      n588 = To Unsigned Byte Integer(number=w868) -> (unsigned 8bit integer=w865:u8)
                      n589 = Add(x=w867, y=w865) -> (x+y=w866:u8)
                      n590 = call "write to RF synth bd.vi"("Address Byte"=w866, "BD 2 Byte"=w869, "BD 1 Byte"=w870) -> ()  [unwired: 2 in]
                    }
                  }
                }
              }
            }
          }
        }
      }
    }
  }
  n591 = node-c288(w5) -> ()
